vi "Cytex.vi"(3 "Xmit Ring":i8=1, 5 "VISA resource name":refnum<visa-resource-name>="GPIB0::7") -> (0 "error out":errorcluster, 2 "dup VISA resource name":refnum<visa-resource-name>)   [LabVIEW 2022 SP3]
uses:
  Motion Controllers/-MotionRoutines/MotionGlobals.vi
panel:
  # "A zero clears all switches. 1-5 selects Xmit ring"
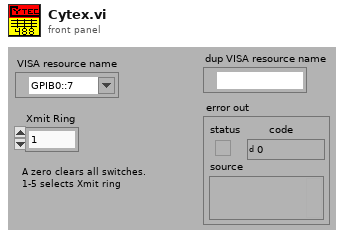
[diagram p1: front panel]
types:
  T1 = typedef "location.ctl" = enum16{"Automatic", "WCM Main", "Hawaii", "Columbia MM3000", "Columbia  NI System", "NYU", "RRI 2", "UHI Allen", "CUMC RT", "Chiba", "Stony Brook", "WCM Microscopy", "WCM Aeoretch", "WCM Optics Lab", "WCM Main 2Axis", "WCM Rotation", "WCM SAM SMAC", "SERI GP"}
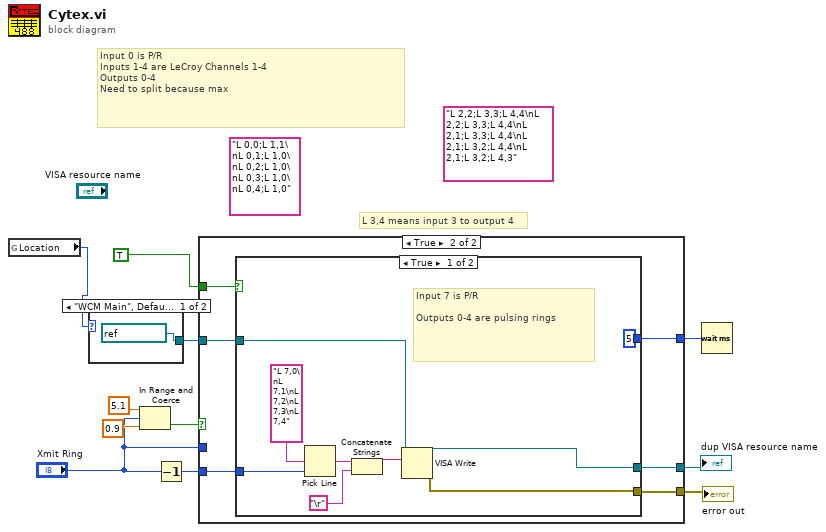
[diagram p0: block diagram]
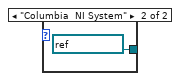
[diagram p2: hidden frame]
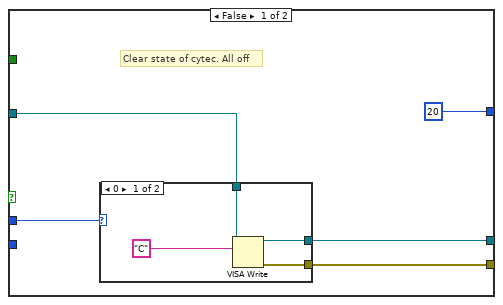
[diagram p3: hidden frame]
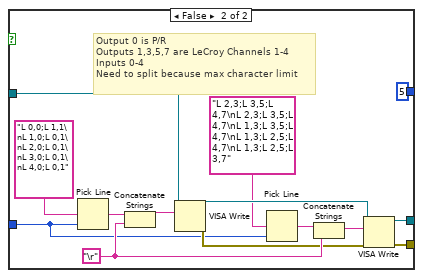
[diagram p5: hidden frame]
diagram:
  (unwired) "L 2,2;L 3,3;L 4,4\nL 2,2;L 3,3;L 4,4\nL 2,1;L 3,3;L 4,4\nL 2,1;L 3,2;L 4,4\nL 2,1;L 3,2;L 4,3"
  (unwired) "L 0,0;L 1,1\nL 0,1;L 1,0\nL 0,2;L 1,0\nL 0,3;L 1,0\nL 0,4;L 1,0"
  # "Input 0 is P/R\nInputs 1-4 are LeCroy Channels 1-4\nOutputs 0-4\nNeed to split because max"
  # "L 3,4 means input 3 to output 4"
  n1 = global read "MotionGlobals.vi" "Location"() -> (w1:T1)
  n2 = case shown="\"WCM Main\", Default" w1 {
    tunnel: [refnum<visa-resource-name> "GPIB::7" ("VISA resource name") refnum<visa-resource-name> "GPIB0::7" ("VISA resource name")] -> w8
    frame "WCM Main", Default {
    }
    frame "Columbia  NI System" {
    }
  }
  n3 = In Range and Coerce(upper limit=5.1, x="Xmit Ring", lower limit=0.9) -> (In Range?=w4:bool)  [unwired: 1 out]
  n4 = Decrement(x="Xmit Ring") -> (x-1=w9:i8)
  n5 = case shown="True" w4 {
    tunnel: w9 -> [_ w26]
    tunnel: [w17 w29] -> w11
    tunnel: [w16 w28] -> w10
    tunnel: w8 -> [w18 w27]
    tunnel: [20 w25] -> w7
    tunnel: "Xmit Ring" -> [w14 _]
    tunnel: TRUE -> [_ w24]
    frame False {
      # "Clear state of cytec. All off"
      n6 = case shown="0" w14 {
        tunnel: w18 -> [w21 w23]
        tunnel: [w20 w23] -> w17
        tunnel: [w19 _] -> w16
        frame 0 {
          n7 = VISA Write(VISA resource name=w21, write buffer="C") -> (VISA resource name out=w20:refnum<visa-resource-name>, error out=w19:errorcluster)  [unwired: 1 in, 1 out]
        }
        frame 1, Default {
        }
      }
    }
    frame True {
      n8 = case shown="True" w24 {
        tunnel: [w31 w45] -> w29
        tunnel: [w30 w44] -> w28
        tunnel: w27 -> [w35 w43]
        tunnel: w26 -> [w34 w42]
        tunnel: [5 5] -> w25
        frame True {
          # "Input 7 is P/R\n\nOutputs 0-4 are pulsing rings"
          n9 = Pick Line(multi-line string="L 7,0\nL 7,1\nL 7,2\nL 7,3\nL 7,4", line index=w34) -> (output string=w37:string)  [unwired: 1 out]
          n10 = Concatenate Strings(w37, "\r") -> (w38:string)
          n11 = VISA Write(VISA resource name=w35, write buffer=w38) -> (VISA resource name out=w31:refnum<visa-resource-name>, error out=w30:errorcluster)  [unwired: 1 in, 1 out]
        }
        frame False {
          w48 = "\r"
          # "Output 0 is P/R\nOutputs 1,3,5,7 are LeCroy Channels 1-4\nInputs 0-4\nNeed to split because max character limit"
          n12 = Pick Line(multi-line string="L 0,0;L 1,1\nL 1,0;L 0,1\nL 2,0;L 0,1\nL 3,0;L 0,1\nL 4,0;L 0,1", line index=w42) -> (output string=w51:string)  [unwired: 1 out]
          n13 = Concatenate Strings(w51, w48) -> (w52:string)
          n14 = VISA Write(VISA resource name=w43, write buffer=w52) -> (VISA resource name out=w47:refnum<visa-resource-name>, error out=w46:errorcluster)  [unwired: 1 in, 1 out]
          n15 = Pick Line(multi-line string="L 2,3;L 3,5;L 4,7\nL 2,3;L 3,5;L 4,7\nL 1,3;L 3,5;L 4,7\nL 1,3;L 2,5;L 4,7\nL 1,3;L 2,5;L 3,7", line index=w42) -> (output string=w49:string)  [unwired: 1 in]
          n16 = Concatenate Strings(w49, w48) -> (w50:string)
          n17 = VISA Write(VISA resource name=w47, write buffer=w50, error in (no error)=w46) -> (VISA resource name out=w45:refnum<visa-resource-name>, error out=w44:errorcluster)  [unwired: 1 out]
        }
      }
    }
  }
  "dup VISA resource name" <- w11
  "error out" <- w10
  n18 = Wait (ms)(milliseconds to wait=w7) -> ()  [unwired: 1 out]
